vi "2D-Array filtern.vi"(7 "Cluster":T1, 9 "2D-String-Array_in":string[][](array[string])=[["45245,25", "Hallo", "Eier"], ["45245,36", "Ballo", "Mehl"], ["45245,84", "Lallo", "Zucker"], ["245", "Trallo", "Salz"], ["45", "Knallo", "Bier"]]) -> (1 "2D-String-Array_gefiltert":string[][](array[string]))   [LabVIEW 2020, in "allgemeine Sub-VIs.lvlib"]
uses:
  allgemeine Sub-VIs.lvlib
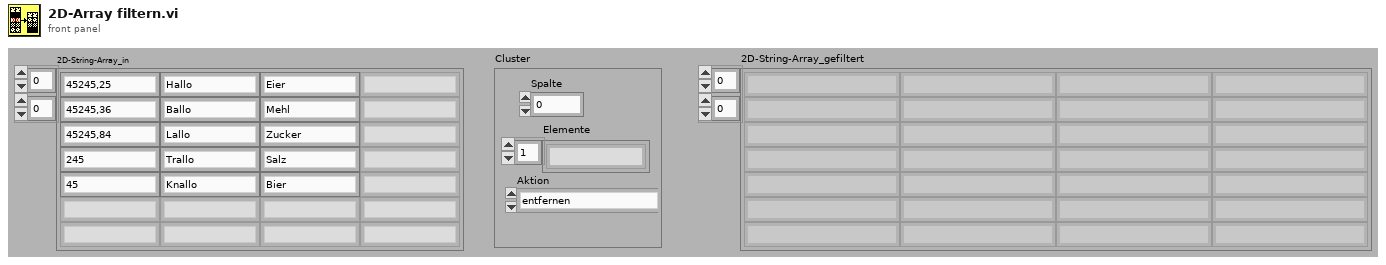
[diagram p1: front panel]
types:
  T1 = cluster{"Spalte":i32, "Elemente":string[], "Aktion":enum16{"entfernen", "nur diese belassen"}}
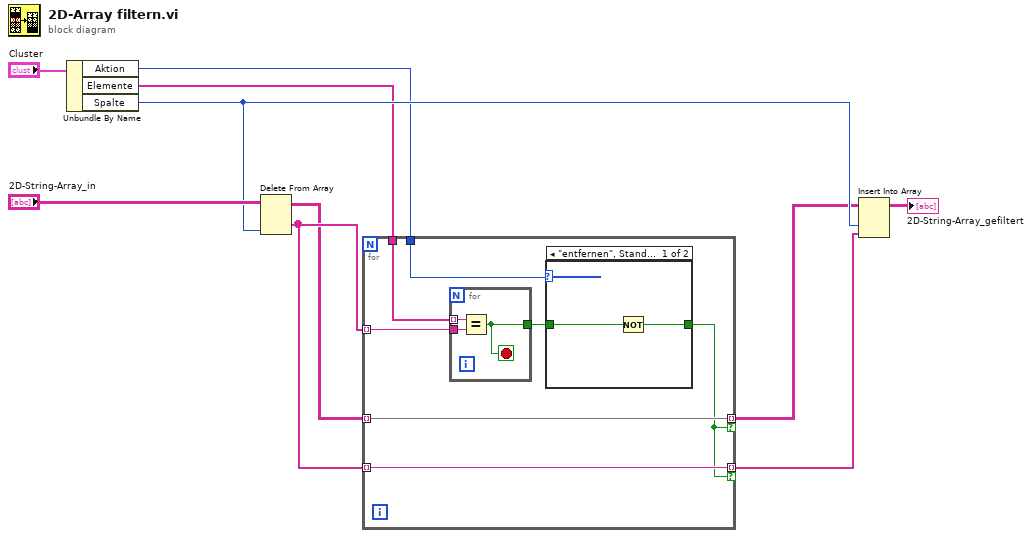
[diagram p0: block diagram]
diagram:
  n1 = Unbundle By Name("Cluster") -> ("Aktion"=w6:enum16{"entfernen", "nur diese belassen"}, "Elemente"=w7:string[], "Spalte"=w8:i32)
  n2 = Delete From Array(array="2D-String-Array_in", index (col)=w8) -> (deleted portion=w5:string[], array with subset deleted=w4:string[][])  [unwired: 2 in]
  n3 = for {
    tunnel: w5 -> [w14] mode=indexing
    tunnel: w7 -> [w17]
    tunnel: w6 -> [w16]
    tunnel: w5 -> [w12] mode=indexing
    tunnel: [w12] -> w2 mode=indexing if=w11
    tunnel: w4 -> [w13] mode=indexing
    tunnel: [w13] -> w3 mode=indexing if=w11
    n4 = for {
      tunnel: w14 -> [w23]
      tunnel: w17 -> [w22] mode=indexing
      tunnel: [w21] -> w15
      stop <- w21 stop-if-true
      n5 = Equal?(x=w22, y=w23) -> (x = y?=w21:bool)
    }
    n6 = case shown="\"entfernen\", Standard" w16 {
      tunnel: w15 -> [w19 w20]
      tunnel: [w18 w20] -> w11
      frame "entfernen", Default {
        n7 = Not(x=w19) -> (.not. x?=w18:bool)
      }
      frame "nur diese belassen" {
      }
    }
  }
  n8 = Insert Into Array(array=w3, index (col)=w8, new element=w2) -> (→"2D-String-Array_gefiltert":string[][])  [unwired: 1 in]
